vi "TempSimV4.vi"() -> ()   [LabVIEW 2021]
uses:
  <vilib>/addons/control/pid/pid.llb/PID (DBL).vi
  <vilib>/addons/control/pid/NI_PID_pid.lvlib
panel:
  in  "PID gains":T1={"proportional gain (Kc)"=1.0, "integral time (Ti, min)"=0.01, "derivative time (Td, min)"=0.0}
  out "T":dbl
  out "Waveform Chart":dbl(graph)
  in  "stop":bool
  in  "Timestep [mS]":dbl
  in  "Tset":dbl
  in  "Tenv":dbl
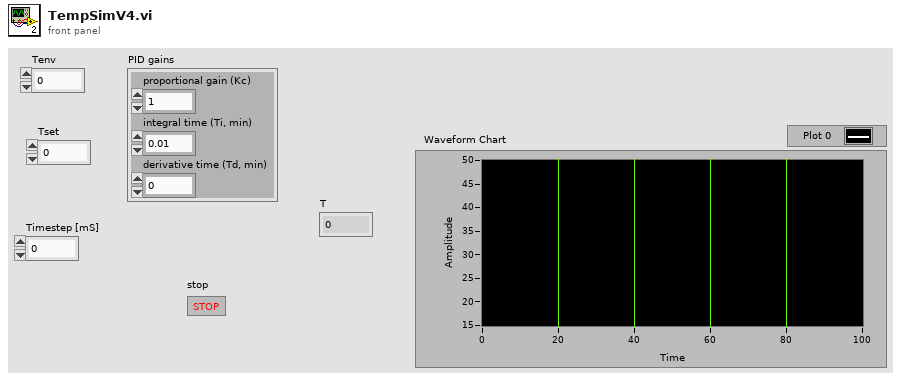
[diagram p1: front panel]
types:
  T1 = cluster{"proportional gain (Kc)":dbl, "integral time (Ti, min)":dbl, "derivative time (Td, min)":dbl}
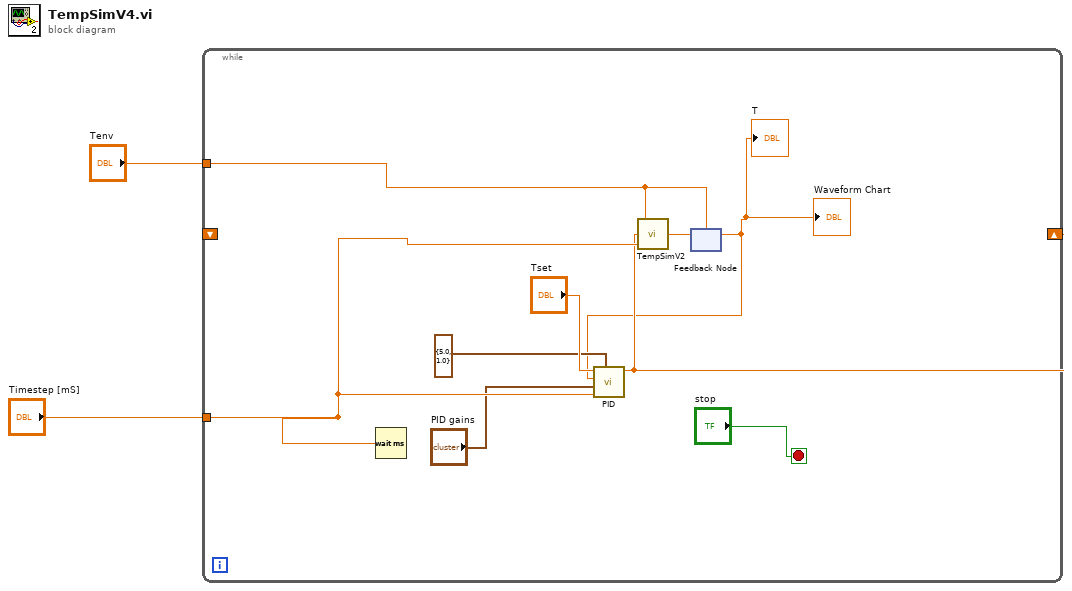
[diagram p0: block diagram]
diagram:
  n1 = while {
    tunnel: "Tenv" -> [w3]
    tunnel: "Timestep [mS]" -> [w10]
    shift-right: [w7] -> _
    shift-left: _ -> [_]
    stop <- "stop" stop-if-true
    n2 = Wait (ms)(milliseconds to wait=w10) -> ()  [unwired: 1 out]
    n3 = feedback #1(w3) -> (w4:dbl)
    "Waveform Chart" <- w4
    "T" <- w4
    n4 = call-poly <vilib>:"PID.vi"("output range"=cluster{"output high":dbl, "output low":dbl} {"output high"=5.0, "output low"=1.0}, "dt (s)"=w10, "PID gains"="PID gains", "process variable"=w4, "setpoint"="Tset") -> ("output"=w7:dbl)  [unwired: 5 in, 1 out]
    n5 = call "TempSimV2.vi"("Timestep [ms]"=w10, "u[V]"=w7, "T_env"=w3) -> ("Tout"=w5:dbl)
    n6 = feedback-in #1(w5) -> ()
  }
